vi "Configure Unit of Voltage.vi"(8 "error in (no error)":errorcluster, 10 "Unit (0: Volts)":u16(ring) items=["Volts", "Watts", "Ohms"], 11 "VISA resource name":refnum<visa-resource-name>) -> (0 "error out":errorcluster, 3 "VISA resource name out":refnum<visa-resource-name>)   [LabVIEW 2017, in "Keithley 2450.lvlib"]
doc: "Configures the voltage measurement units on the instrument."
uses:
  Keithley 2450.lvlib
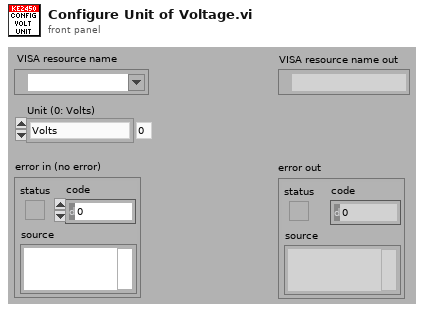
[diagram p1: front panel]
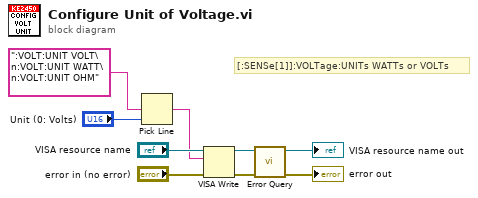
[diagram p0: block diagram]
diagram:
  # "[:SENSe[1]]:VOLTage:UNITs WATTs or VOLTs"
  n1 = Pick Line(multi-line string=":VOLT:UNIT VOLT\n:VOLT:UNIT WATT\n:VOLT:UNIT OHM" ("Function"), line index="Unit (0: Volts)") -> (output string=w1:string)  [unwired: 1 out]
  n2 = VISA Write(VISA resource name="VISA resource name", write buffer=w1, error in (no error)="error in (no error)") -> (VISA resource name out=w3:refnum<visa-resource-name>, error out=w2:errorcluster)  [unwired: 1 out]
  n3 = call "Error Query.vi"("error in (no error)"=w2, "VISA resource name"=w3) -> ("error out"=→"error out":errorcluster, "VISA resource name out"=→"VISA resource name out":refnum<visa-resource-name>)  [unwired: 8 out]
